vi "Intake Rotation Set.vi"() -> ()   [LabVIEW 2017]
uses:
  <vilib>/Rock Robotics/WPI/DriverStation/WPI_DriverStationRobotMode2.ctl
  Intake Rotation Control Type.ctl
  Arm Enum States.ctl
  Intake Rotation Globals.vi
  Robot Global Data.vi
panel:
  out "error out 2":errorcluster
  out "error out":errorcluster
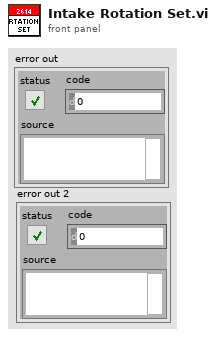
[diagram p1: front panel]
types:
  T1 = typedef "Arm Enum States.ctl" = enum16{"Current Position", "Climb", "Load", "Portal", "Switch", "Scale High", "Scale Mid", "Scale Low", "Exchange", "Stow"}
  T2 = typedef "Intake Rotation Control Type.ctl" = enum16{"No Op", "Manual Up", "Position", "Manual Down", "PositionAuto"}
  T3 = typedef "WPI_DriverStationRobotMode2.ctl" = enum16{"Autonomous Disabled", "Autonomous Enabled", "Teleop Disabled", "Teleop Enabled", "Disconnected", "Finish", "Test Disabled", "Test Enabled", "Emergency Stopped"}
  T4 = typedef "Intake Rotation Notifier.ctl" = cluster{"Step":i32, "Intake Rotation Control Type":T2, "Parameter 1":dbl, "Parameter 2":dbl, "Intake Rotation Notifier":refnum<notifier>, "Manual Up":bool, "Manual Down":bool, "Climb":bool, "Switch":bool, "Scale Low":bool, "Scale High":bool, "Stow":bool, "Load":bool, "Scale Mid":bool, "Exchange":bool, "Set Position":T1, "Portal":bool}
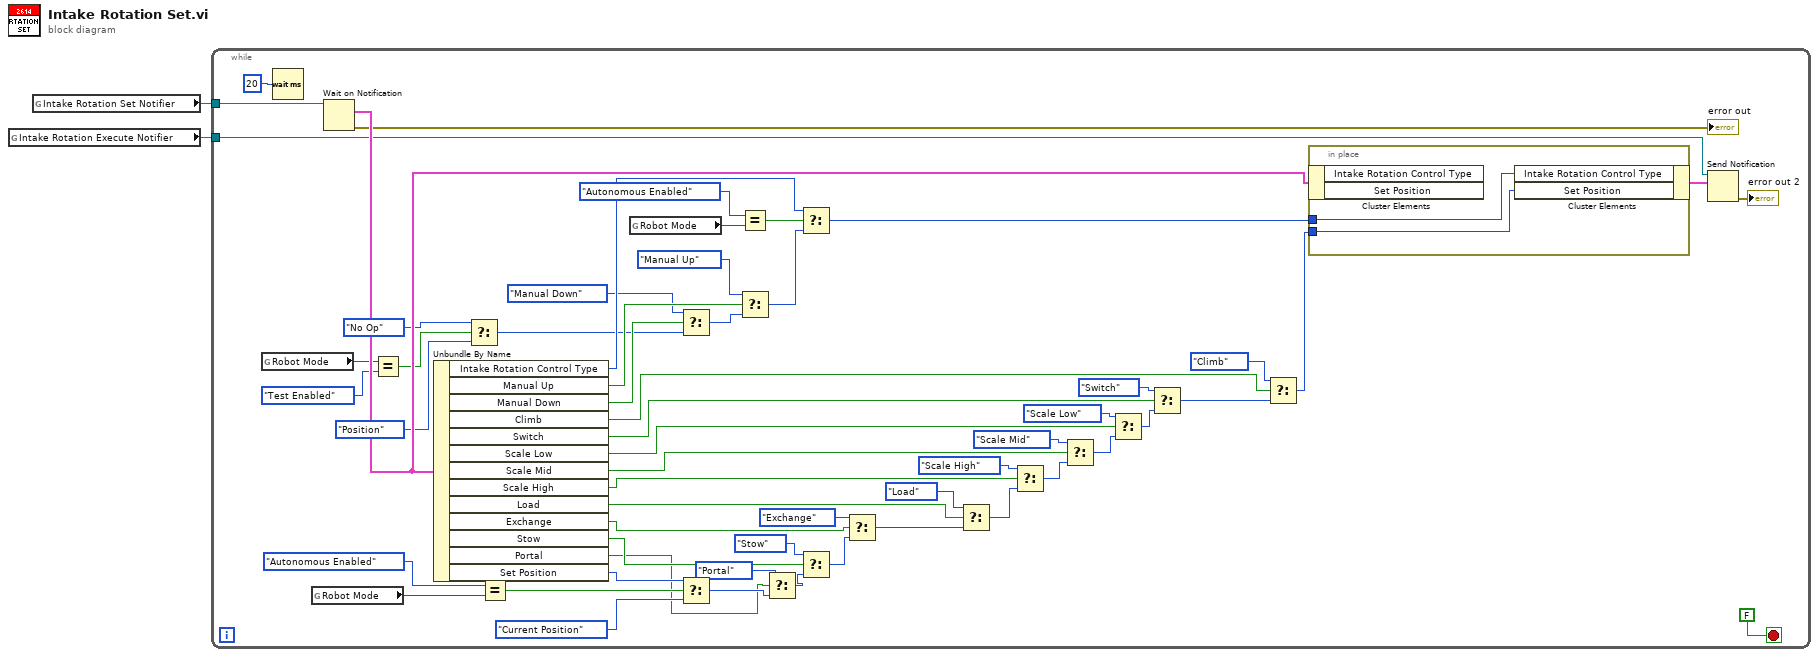
[diagram p0: block diagram]
diagram:
  n1 = global read "Intake Rotation Globals.vi" "Intake Rotation Execute Notifier"() -> (w2:refnum<notifier>)
  n2 = global read "Intake Rotation Globals.vi" "Intake Rotation Set Notifier"() -> (w1:refnum<notifier>)
  n3 = while {
    tunnel: w2 -> [w34]
    tunnel: w1 -> [w33]
    stop <- FALSE stop-if-true
    n4 = global read "Robot Global Data.vi" "Robot Mode"() -> (w31:T3)
    n5 = Wait (ms)(milliseconds to wait=u32 20) -> ()  [unwired: 1 out]
    n6 = global read "Robot Global Data.vi" "Robot Mode"() -> (w23:T3)
    n7 = Wait on Notification(notifier=w33) -> (notification=w57:T4, error out=→"error out":errorcluster)  [unwired: 3 in, 2 out]
    n8 = Equal?(x=w31, y=WPI_DriverStationRobotMode2."Test Enabled") -> (x = y?=w30:bool)
    n9 = Unbundle By Name(w57) -> ("Intake Rotation Control Type"=w55:T2, "Manual Up"=w49:bool, "Manual Down"=w48:bool, "Climb"=w41:bool, "Switch"=w40:bool, "Scale Low"=w39:bool, "Scale Mid"=w38:bool, "Scale High"=w37:bool, "Load"=w36:bool, "Exchange"=w26:bool, "Stow"=w35:bool, "Portal"=w3:bool, "Set Position"=w25:T1)
    n10 = Select(t=Intake_Rotation_Control_Type."No Op" ("Intake Rotation Control Type"), s=w30, f=Intake_Rotation_Control_Type."Position" ("Intake Rotation Control Type")) -> (s? t:f=w32:T2)
    n11 = Equal?(x=WPI_DriverStationRobotMode2."Autonomous Enabled", y=w23) -> (x = y?=w22:bool)
    n12 = global read "Robot Global Data.vi" "Robot Mode"() -> (w53:T3)
    n13 = Select(t=Intake_Rotation_Control_Type."Manual Down", s=w48, f=w32) -> (s? t:f=w50:T2)
    n14 = Select(t=w25, s=w22, f=Arm_Enum_States."Current Position") -> (s? t:f=w5:T1)
    n15 = Equal?(x=WPI_DriverStationRobotMode2."Autonomous Enabled", y=w53) -> (x = y?=w54:bool)
    n16 = Select(t=Intake_Rotation_Control_Type."Manual Up", s=w49, f=w50) -> (s? t:f=w51:T2)
    n17 = Select(t=Arm_Enum_States."Portal", s=w3, f=w5) -> (s? t:f=w6:T1)
    n18 = Select(t=w55, s=w54, f=w51) -> (s? t:f=w56:T2)
    n19 = Select(t=Arm_Enum_States."Stow" ("f"), s=w35, f=w6) -> (s? t:f=w28:T1)
    n20 = Select(t=Arm_Enum_States."Exchange" ("f"), s=w26, f=w28) -> (s? t:f=w27:T1)
    n21 = Select(t=Arm_Enum_States."Load" ("f"), s=w36, f=w27) -> (s? t:f=w42:T1)
    n22 = Select(t=Arm_Enum_States."Scale High" ("f"), s=w37, f=w42) -> (s? t:f=w43:T1)
    n23 = Select(t=Arm_Enum_States."Scale Mid" ("f"), s=w38, f=w43) -> (s? t:f=w44:T1)
    n24 = Select(t=Arm_Enum_States."Scale Low" ("f"), s=w39, f=w44) -> (s? t:f=w45:T1)
    n25 = Select(t=Arm_Enum_States."Switch" ("f"), s=w40, f=w45) -> (s? t:f=w46:T1)
    n26 = Select(t=Arm_Enum_States."Climb" ("f"), s=w41, f=w46) -> (s? t:f=w47:T1)
    n27 = in-place {
      in-place-border: w56 -> [w61]
      in-place-border: w47 -> [w62]
      n28 = in-place-cluster #1(w57) -> ()  [unwired: 2 out]
      n29 = in-place-cluster #1("Intake Rotation Control Type"=w61, "Set Position"=w62) -> (w58:T4)
    }
    n30 = Send Notification(notification=w58, notifier=w34) -> (error out=→"error out 2":errorcluster)  [unwired: 1 in, 1 out]
  }
